vi "Add New Request.vi"(8 "Error In":errorcluster) -> (0 "Error Out":errorcluster)   [LabVIEW 2015]
uses:
  LVClasses/Request/PersonnelType.ctl
  LVClasses/Request/RequestType.ctl
  LVClasses/Personnel/Personnel.lvclass/Personnel.ctl
  LVClasses/Personnel/Read Name.vi
  LVClasses/Personnel/Read Role.vi
  LVClasses/Personnel/Read UniqueID.vi
  LVRestAPI/RoomRestApi.lvlib
  LVClasses/Request/Request.lvclass
  LVRestAPI/PersonnelRestApi.lvlib
  LVClasses/Personnel/Personnel.lvclass
panel:
  in  "Personnel Name":u16(ring) items=["A", "B", "C", "D"]
  in  "Submit":bool
  in  "Cancel":bool
  in  "Room":i32
  in  "Request Type":T1
  in  "Personnel Type":T2 items=["Nurse", "Doctor", "Cleanning", "Admin"]
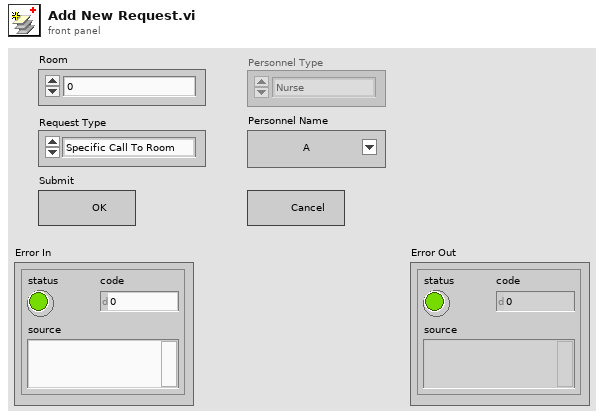
[diagram p1: front panel]
types:
  T1 = typedef "Request.lvclass/RequestType.ctl" = enum16{"Specific Call To Room", "General Call To Room"}
  T2 = typedef "Request.lvclass/PersonnelType.ctl" = u16
  T3 = enum8{"Enabled", "Disabled", "Disabled and Grayed Out"}
  T4 = typedef "Personnel.lvclass/PersonnelType.ctl" = enum16{"Nurse", "Doctor", "Cleanning", "Admin"}
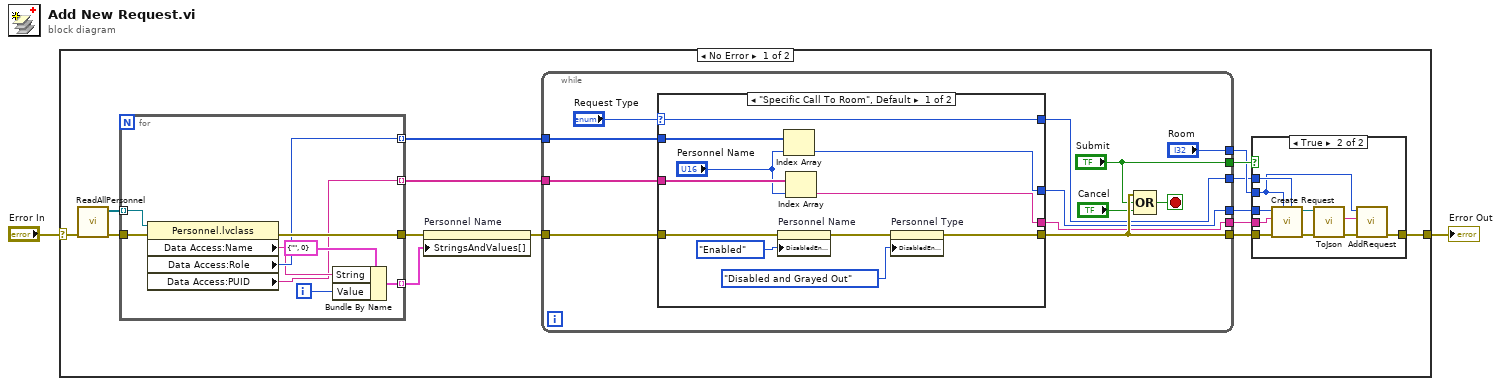
[diagram p0: block diagram]
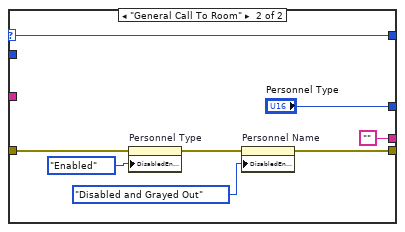
[diagram p3: hidden frame]
diagram:
  n1 = case shown="No Error" "Error In" {
    selector: "Error In" -> [w17 w69]
    tunnel: [w14 w69] -> w1
    frame No Error {
      n2 = call "ReadAllPersonnel.vi"("error in (no error)"=w17) -> ("error out"=w8:errorcluster, "Personnel"=w10:refnum<class "Personnel.lvclass">[])  [unwired: 7 in, 2 out]
      n3 = for {
        tunnel: w10 -> [w26] mode=indexing
        tunnel: w8 -> [w25]
        tunnel: [w24] -> w7
        tunnel: [w23] -> w5 mode=indexing
        tunnel: [w20] -> w4 mode=indexing
        tunnel: [w18] -> w3 mode=indexing
        i -> [w21]
        n4 = property class="Personnel.lvclass"(reference=w26, error in=w25) -> (error out=w24:errorcluster, "Data Access:Name"=w19:string, "Data Access:Role"=w20:T4, "Data Access:PUID"=w18:string)  [unwired: 1 out]
        n5 = Bundle By Name(cluster=cluster{"String":string, "Value":u16} {"String"="", "Value"=0}, "String"=w19, "Value"=w21) -> (w23:cluster{"String":string, "Value":u16})
      }
      n6 = property on="Personnel Name" class="Ring (strict)"(error in=w7, "StringsAndValues[]"=w5) -> (error out=w9:errorcluster)  [unwired: 1 in, 1 out]
      n7 = while {
        tunnel: w9 -> [w48]
        tunnel: [w46] -> w15
        tunnel: ["Submit"] -> w16
        tunnel: ["Room"] -> w13
        tunnel: [w42] -> w12
        tunnel: [w41] -> w11
        tunnel: [w40] -> w6
        tunnel: w4 -> [w39]
        tunnel: w3 -> [w38]
        stop <- w47 stop-if-true
        n8 = case shown="\"Specific Call To Room\", Default" "Request Type" {
          selector: "Request Type" -> [w60 w67]
          tunnel: w48 -> [w57 w68]
          tunnel: [w59 w64] -> w46
          tunnel: [w60 w67] -> w42
          tunnel: [w51 ""] -> w41
          tunnel: [w54 "Personnel Type"] -> w40
          tunnel: w39 -> [w53 _]
          tunnel: w38 -> [w52 _]
          frame "Specific Call To Room", Default {
            n9 = property on="Personnel Name" class="Ring (strict)"(error in=w57, "DisabledEnum"=T3."Enabled" ("Disabled")) -> (error out=w56:errorcluster)  [unwired: 1 in, 1 out]
            n10 = Index Array(array=w53, index="Personnel Name") -> (element=w54:T4)
            n11 = Index Array(array=w52, index="Personnel Name") -> (element=w51:string)
            n12 = property on="Personnel Type" class="Ring (strict)"(error in=w56, "DisabledEnum"=T3."Disabled and Grayed Out" ("Disabled")) -> (error out=w59:errorcluster)  [unwired: 1 in, 1 out]
          }
          frame "General Call To Room" {
            n13 = property on="Personnel Type" class="Ring (strict)"(error in=w68, "DisabledEnum"=T3."Enabled" ("Disabled")) -> (error out=w65:errorcluster)  [unwired: 1 in, 1 out]
            n14 = property on="Personnel Name" class="Ring (strict)"(error in=w65, "DisabledEnum"=T3."Disabled and Grayed Out" ("Disabled")) -> (error out=w64:errorcluster)  [unwired: 1 in, 1 out]
          }
        }
        n15 = Compound Arithmetic op=OR(w46, "Submit", "Cancel") -> (w47:bool)
      }
      n16 = case shown="True" w16 {
        tunnel: w15 -> [w27 w37]
        tunnel: [w27 w32] -> w14
        tunnel: w13 -> [_ w31]
        tunnel: w12 -> [_ w34]
        tunnel: w11 -> [_ w28]
        tunnel: w6 -> [_ w29]
        frame False {
        }
        frame True {
          n17 = call "Create Request.vi"("Request Type"=w34, "Room Number"=w31, "error in (no error)"=w37, "Name"=w28, "Personnel Type"=w29) -> ("error out"=w36:errorcluster, "Request out"=w35:refnum<class "Request.lvclass">)  [unwired: 4 in, 1 out]
          n18 = call "ToJson.vi"("error in (no error)"=w36, "Request"=w35) -> ("error out"=w33:errorcluster, "Request"=w30:string)  [unwired: 8 in]
          n19 = call "AddRequest.vi"("error in (no error)"=w33, "Request"=w30, "Room Number"=w31) -> ("error out"=w32:errorcluster)  [unwired: 7 in, 1 out]
        }
      }
    }
    frame Error {
    }
  }
  "Error Out" <- w1
